vi "MGCC_FntStaMach_main_PhaseTwo.vi"() -> ()   [LabVIEW 2016]
uses:
  Sub-VIs/MGCC_FntStaMach_gobal.vi
  Communication/Global communication.vi
  <vilib>/Utility/error.llb/Error Cluster From Error Code.vi
  Abnormal Fault State Control/Sub_VIs/Fault_Abnormal_state.vi
  <vilib>/ErrorRing/Error Ring.xnode
panel:
  in  "b_MGCC_FntStaMach_Event_Manually_Control":bool
  out "Next_States":string[](array[string])
  out "Next_node":dbl[](array[numeric])
  out "Error output":errorcluster[](array[cluster])
  # "Copyright <2020> <The University of Tennessee at Knoxville and the University of Tennessee Research Foundation>\n\nRedistribution and use in source and binary forms, with or without modification, are permitted provided that the following conditions are met:\n\n1. Redistributions of source code must retain the above copyright notice, this list of conditions and the following disclaimer.\n\n2. Redistributions in binary form must reproduce the above copyright notice, this list of conditions and the following disclaimer in the documentation and/or other materials provided with the distribution.\n\n3. Neither the name of the copyright holder nor the names of its contributors may be used to endorse or promote products derived from this software without specific prior written permission.\n\nTHIS SOFTWARE IS PROVIDED BY THE COPYRIGHT HOLDERS AND CONTRIBUTORS \"AS IS\" AND ANY EXPRESS OR IMPLIED WARRANTIES, INCLUDING, BUT NOT LIMITED TO, THE IMPLIED WARRANTIES OF MERCHANTABILITY AND FITNESS FOR A PARTICULAR PURPOSE ARE DISCLAIMED. IN NO EVENT SHALL THE COPYRIGHT HOLDER OR CONTRIBUTORS BE LIABLE FOR ANY DIRECT, INDIRECT, INCIDENTAL, SPECIAL, EXEMPLARY, OR CONSEQUENTIAL DAMAGES (INCLUDING, BUT NOT LIMITED TO, PROCUREMENT OF SUBSTITUTE GOODS OR SERVICES; LOSS OF USE, DATA, OR PROFITS; OR BUSINESS INTERRUPTION) HOWEVER CAUSED AND ON ANY THEORY OF LIABILITY, WHETHER IN CONTRACT, STRICT LIABILITY, OR TORT (INCLUDING NEGLIGENCE OR OTHERWISE) ARISING IN ANY WAY OUT OF THE USE OF THIS SOFTWARE, EVEN IF ADVISED OF THE POSSIBILITY OF SUCH DAMAGE."
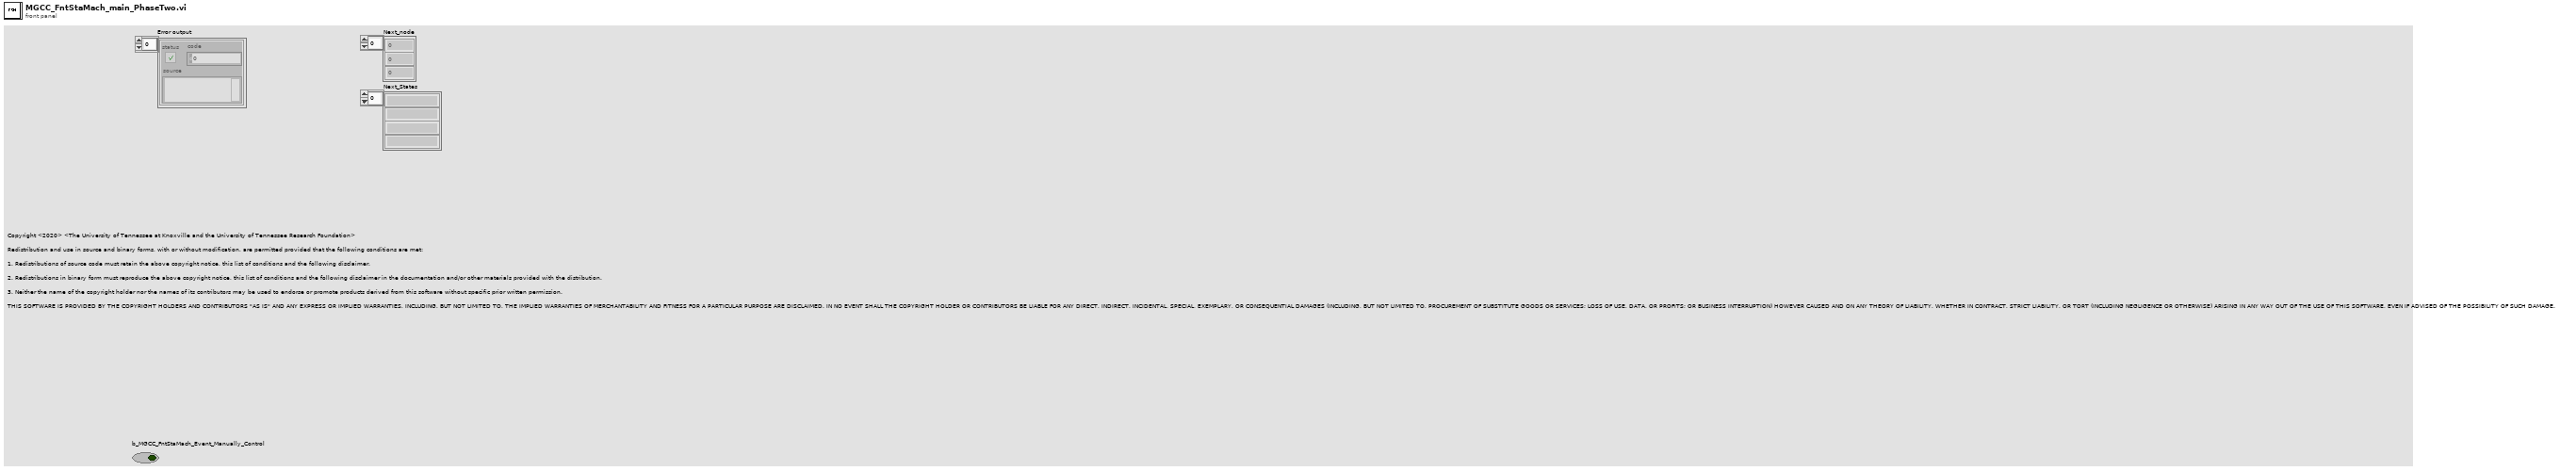
[diagram p1: front panel]
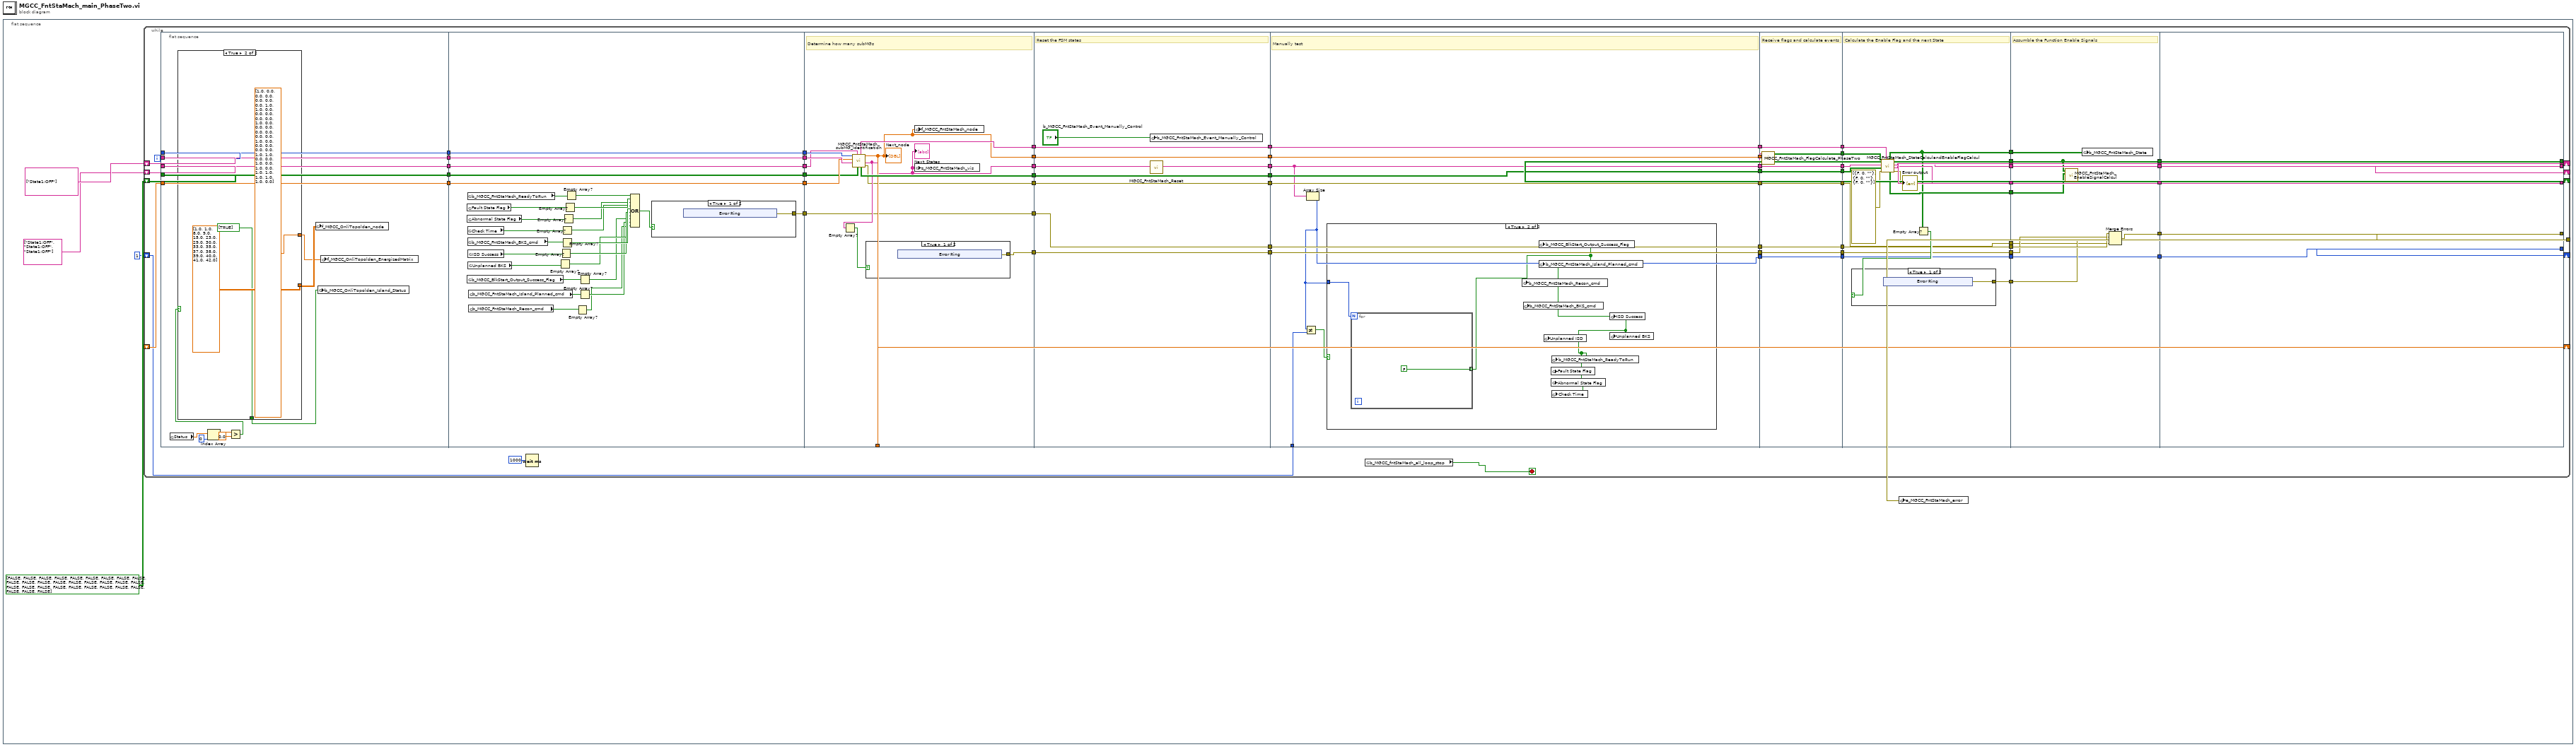
[diagram p0: block diagram]
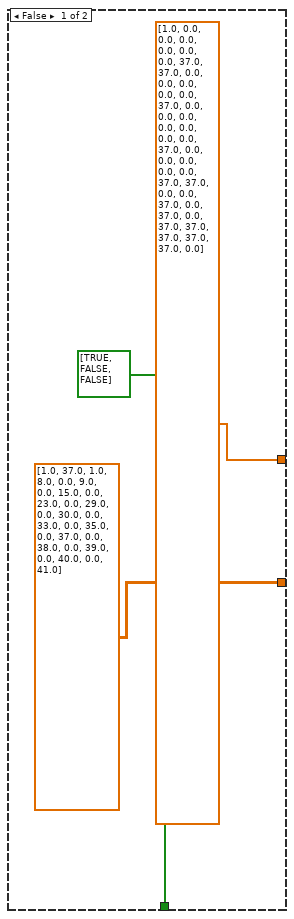
[diagram p2: hidden frame]
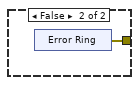
[diagram p3: hidden frame]
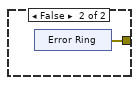
[diagram p4: hidden frame]
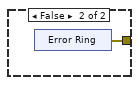
[diagram p6: hidden frame]
diagram:
  n1 = flat-sequence {
    frame #0 {
      n2 = while {
        shift-right: [w71] -> _
        shift-left: string[] ["State1:OFF"] ("Output State") -> [w74]
        shift-right: [w70] -> _
        shift-left: string[] ["State1:OFF", "State1:OFF", "State1:OFF"] ("ABN State output") -> [w58]
        shift-right: [w69] -> _
        shift-left: bool[][] [[FALSE, FALSE, FALSE, FALSE, FALSE, FALSE, FALSE, FALSE, FALSE, FALSE], [FALSE, FALSE, FALSE, FALSE, FALSE, FALSE, FALSE, FALSE, FALSE, FALSE], [FALSE, FALSE, FALSE, FALSE, FALSE, FALSE, FALSE, FALSE, FALSE, FALSE]] ("ABN Function Enable output") -> [w57]
        shift-right: [w62] -> _
        shift-left: _ -> [w61]
        tunnel: [w22] -> w2
        shift-right: [w12] -> _
        shift-left: 1 -> [w11]
        i -> [w60]
        stop <- w17 stop-if-true
        n3 = flat-sequence {
          tunnel: w57 -> [w84]
          tunnel: w58 -> [w85]
          tunnel: w60 -> [w86]
          tunnel: w61 -> [w87]
          tunnel: w74 -> [w88]
          tunnel: [w88] -> w10
          tunnel: [w87] -> w9
          tunnel: [w86] -> w8
          tunnel: [w85] -> w7
          tunnel: [w84] -> w6
          tunnel: [w121] -> w44
          tunnel: [w120] -> w43
          tunnel: [w119] -> w42
          tunnel: [w118] -> w41
          tunnel: [w117] -> w40
          tunnel: [w95] -> w34
          tunnel: w10 -> [w121]
          tunnel: w9 -> [w120]
          tunnel: w8 -> [w119]
          tunnel: w7 -> [w118]
          tunnel: w6 -> [w117]
          tunnel: [w134] -> w63
          tunnel: [w135] -> w62
          tunnel: [w135] -> w59
          tunnel: [w137] -> w55
          tunnel: [w136] -> w53
          tunnel: w44 -> [w142]
          tunnel: w43 -> [w141]
          tunnel: w42 -> [w140]
          tunnel: w41 -> [w139]
          tunnel: w40 -> [w138]
          tunnel: [w132] -> w35
          tunnel: w34 -> [w132]
          tunnel: [w131] -> w29
          tunnel: [w130] -> w23
          tunnel: [w159] -> w52
          tunnel: w63 -> [w157]
          tunnel: [w158] -> w50
          tunnel: w59 -> [w158]
          tunnel: [w156] -> w48
          tunnel: w55 -> [w156]
          tunnel: [w155] -> w46
          tunnel: w53 -> [w155]
          tunnel: [w153] -> w36
          tunnel: w35 -> [w153]
          tunnel: [w152] -> w30
          tunnel: w29 -> [w152]
          tunnel: [w151] -> w24
          tunnel: w23 -> [w151]
          tunnel: w52 -> [w163]
          tunnel: [w163] -> w51
          tunnel: w50 -> [w169]
          tunnel: [w169] -> w49
          tunnel: w48 -> [w168]
          tunnel: [w168] -> w47
          tunnel: w46 -> [w167]
          tunnel: [w167] -> w45
          tunnel: [w166] -> w37
          tunnel: w36 -> [w166]
          tunnel: [w165] -> w31
          tunnel: w30 -> [w165]
          tunnel: [w164] -> w25
          tunnel: w24 -> [w164]
          tunnel: [w160] -> w13
          tunnel: w11 -> [w162]
          tunnel: w51 -> [w180]
          tunnel: [w181] -> w73
          tunnel: [w180] -> w72
          tunnel: w49 -> [w179]
          tunnel: [w178] -> w56
          tunnel: w47 -> [w178]
          tunnel: [w177] -> w54
          tunnel: w45 -> [w177]
          tunnel: [w176] -> w38
          tunnel: w37 -> [w176]
          tunnel: [w175] -> w32
          tunnel: w31 -> [w175]
          tunnel: [w174] -> w26
          tunnel: w25 -> [w174]
          tunnel: [w173] -> w14
          tunnel: w13 -> [w173]
          tunnel: w73 -> [w198]
          tunnel: w72 -> [w197]
          tunnel: [w196] -> w68
          tunnel: [w195] -> w67
          tunnel: [w194] -> w66
          tunnel: [w188] -> w65
          tunnel: [w191] -> w64
          tunnel: w56 -> [w190]
          tunnel: w54 -> [w189]
          tunnel: [w186] -> w39
          tunnel: w38 -> [w186]
          tunnel: [w185] -> w33
          tunnel: w32 -> [w185]
          tunnel: [w184] -> w28
          tunnel: [w183] -> w27
          tunnel: w26 -> [w183]
          tunnel: [w182] -> w15
          tunnel: w14 -> [w182]
          tunnel: w68 -> [w217]
          tunnel: w67 -> [w216]
          tunnel: w66 -> [w214]
          tunnel: w65 -> [w215]
          tunnel: w64 -> [w213]
          tunnel: w39 -> [w212]
          tunnel: w33 -> [w211]
          tunnel: w28 -> [w210]
          tunnel: w27 -> [w209]
          tunnel: [w217] -> w21
          tunnel: [w216] -> w20
          tunnel: [w214] -> w19
          tunnel: [w208] -> w18
          tunnel: [w207] -> w16
          tunnel: w15 -> [w207]
          tunnel: [w220] -> w22
          tunnel: [w221] -> w69
          tunnel: [w222] -> w70
          tunnel: [w219] -> w71
          tunnel: w21 -> [w219]
          tunnel: w20 -> [w222]
          tunnel: w19 -> [w221]
          tunnel: w18 -> [w220]
          tunnel: [w218] -> w12
          tunnel: w16 -> [w218]
          frame #0 {
            n4 = global read "Global communication.vi" "Status"() -> (w82:dbl[])
            n5 = Index Array(array=w82, index=0) -> (element=w80:dbl)
            n6 = Greater?(x=w80, y=0.0) -> (0:w78:bool)
            n7 = case shown="True" w78 {
              tunnel: [dbl[][] [[1.0, 37.0], [1.0, 8.0], [0.0, 9.0], [0.0, 15.0], [0.0, 23.0], [0.0, 29.0], [0.0, 30.0], [0.0, 33.0], [0.0, 35.0], [0.0, 37.0], [0.0, 38.0], [0.0, 39.0], [0.0, 40.0], [0.0, 41.0]] dbl[][] [[1.0], [1.0], [8.0], [9.0], [15.0], [23.0], [29.0], [30.0], [33.0], [35.0], [37.0], [38.0], [39.0], [40.0], [41.0], [42.0]]] -> w83
              tunnel: [dbl[] [1.0, 0.0, 0.0, 0.0, 0.0, 0.0, 0.0, 37.0, 37.0, 0.0, 0.0, 0.0, 0.0, 0.0, 37.0, 0.0, 0.0, 0.0, 0.0, 0.0, 0.0, 0.0, 37.0, 0.0, 0.0, 0.0, 0.0, 0.0, 37.0, 37.0, 0.0, 0.0, 37.0, 0.0, 37.0, 0.0, 37.0, 37.0, 37.0, 37.0, 37.0, 0.0] dbl[] [1.0, 0.0, 0.0, 0.0, 0.0, 0.0, 0.0, 1.0, 1.0, 0.0, 0.0, 0.0, 0.0, 0.0, 1.0, 0.0, 0.0, 0.0, 0.0, 0.0, 0.0, 0.0, 1.0, 0.0, 0.0, 0.0, 0.0, 0.0, 1.0, 1.0, 0.0, 0.0, 1.0, 0.0, 1.0, 0.0, 1.0, 1.0, 1.0, 1.0, 1.0, 0.0]] -> w77
              tunnel: [bool[] [TRUE, FALSE, FALSE] bool[] [TRUE]] -> w76
              frame False {
              }
              frame True {
              }
            }
            n8 = global write "MGCC_FntStaMach_gobal.vi" "f_MGCC_OnliTopolden_node"(w83) -> ()
            n9 = global write "MGCC_FntStaMach_gobal.vi" "b_MGCC_OnliTopolden_Island_Status"(w76) -> ()
            n10 = global write "MGCC_FntStaMach_gobal.vi" "f_MGCC_OnliTopolden_EnergizedMatrix"(w77) -> ()
          }
          frame #1 {
            n11 = global read "MGCC_FntStaMach_gobal.vi" "Fault State Flag"() -> (w115:bool[])
            n12 = global read "MGCC_FntStaMach_gobal.vi" "Abnormal State Flag"() -> (w114:bool[])
            n13 = global read "MGCC_FntStaMach_gobal.vi" "b_MGCC_BlkStart_Output_Success_Flag"() -> (w109:bool[])
            n14 = global read "MGCC_FntStaMach_gobal.vi" "b_MGCC_FntStaMach_ReadyToRun"() -> (w116:bool[])
            n15 = global read "MGCC_FntStaMach_gobal.vi" "Check Time"() -> (w113:bool[])
            n16 = global read "MGCC_FntStaMach_gobal.vi" "b_MGCC_FntStaMach_BKS_cmd"() -> (w112:bool[])
            n17 = global read "MGCC_FntStaMach_gobal.vi" "ISD Success"() -> (w111:bool[])
            n18 = global read "MGCC_FntStaMach_gobal.vi" "Unplanned BKS"() -> (w110:bool[])
            n19 = global read "MGCC_FntStaMach_gobal.vi" "b_MGCC_FntStaMach_Island_Planned_cmd"() -> (w108:bool[])
            n20 = global read "MGCC_FntStaMach_gobal.vi" "b_MGCC_FntStaMach_Recon_cmd"() -> (w107:bool[])
            n21 = Empty Array?(array=w110) -> (empty?=w100:bool)
            n22 = Empty Array?(array=w111) -> (empty?=w101:bool)
            n23 = Empty Array?(array=w113) -> (empty?=w103:bool)
            n24 = Empty Array?(array=w112) -> (empty?=w102:bool)
            n25 = Empty Array?(array=w114) -> (empty?=w104:bool)
            n26 = Empty Array?(array=w115) -> (empty?=w105:bool)
            n27 = Empty Array?(array=w116) -> (empty?=w106:bool)
            n28 = Empty Array?(array=w107) -> (empty?=w97:bool)
            n29 = Empty Array?(array=w109) -> (empty?=w99:bool)
            n30 = Empty Array?(array=w108) -> (empty?=w98:bool)
            n31 = Compound Arithmetic op=OR(w106, w105, w104, w103, w102, w101, w100, w99, w98, w97) -> (w96:bool)
            n32 = case shown="True" w96 {
              tunnel: [w122 w128] -> w95
              frame True {
                n33 = xnode "Error Ring"() -> ("error out"=w122:errorcluster)
              }
              frame False {
                n34 = xnode "Error Ring"() -> ("error out"=w128:errorcluster)
              }
            }
          }
          frame #2 {
            # "Determine how many subMGs"
            n35 = call "MGCC_FntStaMach_subMG_Identification.vi"("Abnormal_enable_input"=w138, "Abnormal input"=w139, "Previous_states 2"=w142, "Previous_node"=w141, "Turns"=w140) -> ("error out 2"=w130:errorcluster, "Next_States"=w134:string[], "Next_node"=w135:dbl[], "Abnormal_enable_output"=w136:bool[][], "Abnormal_output"=w137:string[])  [unwired: 2 in]
            "Next_node" <- w135
            "Next_States" <- w134
            n36 = Empty Array?(array=w134) -> (empty?=w133:bool)
            n37 = case shown="True" w133 {
              tunnel: [w143 w149] -> w131
              frame True {
                n38 = xnode "Error Ring"() -> ("error out"=w143:errorcluster)
              }
              frame False {
                n39 = xnode "Error Ring"() -> ("error out"=w149:errorcluster)
              }
            }
            n40 = global write "MGCC_FntStaMach_gobal.vi" "f_MGCC_FntStaMach_node"(w135) -> ()
            n41 = global write "MGCC_FntStaMach_gobal.vi" "s_MGCC_FntStaMach_vis"(w134) -> ()
          }
          frame #3 {
            # "Reset the FSM states"
            n42 = global write "MGCC_FntStaMach_gobal.vi" "b_MGCC_FntStaMach_Event_Manually_Control"("b_MGCC_FntStaMach_Event_Manually_Control") -> ()
            n43 = call "MGCC_FntStaMach_Reset.vi"("Input State"=w157) -> ("Output State"=w159:string[])  [unwired: 10 in]
          }
          frame #4 {
            # "Manually test"
            n44 = Array Size(array=w163) -> (size(s)=w160:i32)
            n45 = Not Equal?(x=w160, y=w162) -> (x != y?=w161:bool)
            n46 = case shown="True" w161 {
              tunnel: w160 -> [_ w170]
              frame False {
              }
              frame True {
                n47 = for {
                  N: w170 -> [_]
                  tunnel: [FALSE ("b_MGCC_FntStaMach_ReadyToRun")] -> w171 mode=indexing
                }
                n48 = global write "MGCC_FntStaMach_gobal.vi" "b_MGCC_FntStaMach_Recon_cmd"(w171) -> ()
                n49 = global write "MGCC_FntStaMach_gobal.vi" "b_MGCC_FntStaMach_BKS_cmd"(w171) -> ()
                n50 = global write "MGCC_FntStaMach_gobal.vi" "b_MGCC_BlkStart_Output_Success_Flag"(w171) -> ()
                n51 = global write "MGCC_FntStaMach_gobal.vi" "b_MGCC_FntStaMach_Island_Planned_cmd"(w171) -> ()
                n52 = global write "MGCC_FntStaMach_gobal.vi" "Unplanned ISD"(w171) -> ()
                n53 = global write "MGCC_FntStaMach_gobal.vi" "Fault State Flag"(w171) -> ()
                n54 = global write "MGCC_FntStaMach_gobal.vi" "Abnormal State Flag"(w171) -> ()
                n55 = global write "MGCC_FntStaMach_gobal.vi" "b_MGCC_FntStaMach_ReadyToRun"(w171) -> ()
                n56 = global write "MGCC_FntStaMach_gobal.vi" "Check Time"(w171) -> ()
                n57 = global write "MGCC_FntStaMach_gobal.vi" "ISD Success"(w171) -> ()
                n58 = global write "MGCC_FntStaMach_gobal.vi" "Unplanned BKS"(w171) -> ()
              }
            }
          }
          frame #5 {
            # "Receive flags and calculate events"
            n59 = call "MGCC_FntStaMach_FlagCalculate_PhaseTwo.vi"("Current SubMG"=w179, "Input State"=w180) -> ("Output Event"=w181:bool[][])  [unwired: 9 in]
          }
          frame #6 {
            # "Calculate the Enable Flag and the next State"
            n60 = call "MGCC_FntStaMach_StateCalculandEnableFlagCalcul.vi"("ABN State Input"=w190, "Error Input"=errorcluster[] [{"status"=FALSE, "code"=0, "source"=""}, {"status"=FALSE, "code"=0, "source"=""}, {"status"=FALSE, "code"=0, "source"=""}], "ABN State input enable"=w189, "Current State"=w197, "Input Events"=w198) -> ("Error output"=→"Error output":errorcluster[], "Next State"=w196:string[], "ABN State output"=w195:string[], "ABN Function Enable output"=w194:bool[][], "Function Enable 2"=w191:bool[][], "Function Enable 1"=w188:bool[][])  [unwired: 1 in]
            n61 = Empty Array?(array=w188) -> (empty?=w187:bool)
            n62 = case shown="True" w187 {
              tunnel: [w199 w205] -> w184
              frame True {
                n63 = xnode "Error Ring"() -> ("error out"=w199:errorcluster)
              }
              frame False {
                n64 = xnode "Error Ring"() -> ("error out"=w205:errorcluster)
              }
            }
          }
          frame #7 {
            # "Assumble the Function Enable Signals"
            n65 = call "MGCC_FntStaMach_EnableSignalCalcul.vi"("Input enable 2"=w213, "Input enable 1"=w214) -> ()  [unwired: 10 in]
            n66 = global write "MGCC_FntStaMach_gobal.vi" "b_MGCC_FntStaMach_State"(w215) -> ()
            n67 = Merge Errors(w212, w211, w210, w209) -> (w208:errorcluster)
          }
          frame #8 {
          }
        }
        n68 = Wait (ms)(milliseconds to wait=u32 1000) -> ()  [unwired: 1 out]
        n69 = global read "MGCC_FntStaMach_gobal.vi" "b_MGCC_fntStaMach_all_loop_stop"() -> (w17:bool)
      }
      n70 = global write "Fault_Abnormal_state.vi" "e_MGCC_FntStaMach_error"(w2) -> ()
    }
  }
